vi "Controller Process.vi"(8 "error in (no error)":errorcluster, 11 "View Model":T1) -> (0 "error out":errorcluster)   [LabVIEW 2017]
doc: "The SW component that allows the user to interact with the controls and provides appropriate feedback."
uses:
  Model/Controls/View Model.ctl
  Model/Controls/Shared Model.ctl
  Error Handler/Controls/Error Model.ctl
  Error Handler/Controls/Error Message.ctl
  Error Handler/Controls/Error Type.ctl
  Configuration/Controls/Config Model.ctl
  Configuration/Controls/Config DB Message.ctl
  Configuration/Controls/Config DB Command.ctl
  Configuration/Controls/Config DB Overhead.ctl
  Configuration/Controls/Config DB Record.ctl
  Controls/Controller Model.ctl
  Views/Vehicle Position Simulation View/Controls/Vehicle - Position.ctl
  Controls/Controller Overhead.ctl
  Controls/Controller Wash Step.ctl
  Controls/Controller State.ctl
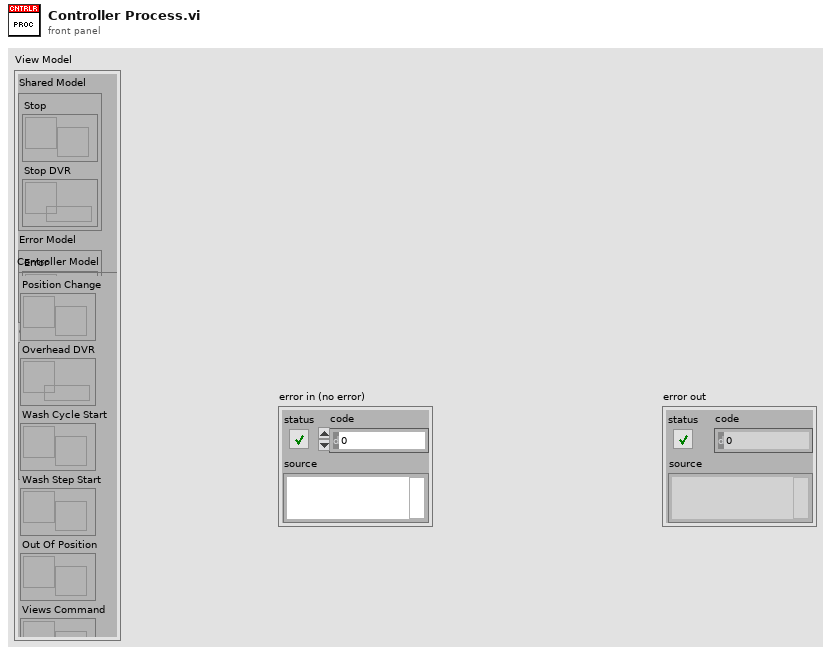
[diagram p1: front panel]
types:
  T1 = typedef "View Model.ctl" = cluster{"Shared Model":T2, "Error Model":T3, "Config Model":T4, "Controller Model":T5}
  T2 = typedef "Shared Model.ctl" = cluster{"Stop":refnum<user-event>, "Stop DVR":refnum<data-value>}
  T3 = typedef "Error Model.ctl" = cluster{"Error":refnum<user-event>}
  T4 = typedef "Config Model.ctl" = cluster{"Config":refnum<user-event>, "Config DVR":refnum<data-value>}
  T5 = typedef "Controller Model.ctl" = cluster{"Position Change":refnum<user-event>, "Overhead DVR":refnum<data-value>, "Wash Cycle Start":refnum<user-event>, "Wash Step Start":refnum<user-event>, "Out Of Position":refnum<user-event>, "Views Command":refnum<user-event>}
  T6 = typedef "Controller State.ctl" = enum16{"Initial", "Wait for Start", "Wash Cycle Start", "Wash Cycle Complete", "Wash Step Start", "Wash Step Execute", "Wash Step Complete", "Wait for Vehicle Position", "Wash Exit", "Wash Abort/Terminate"}
  T7 = typedef "Error Type.ctl" = enum16{"Minor Error", "Wash Cycle Error", "System Error", "Unknown"}
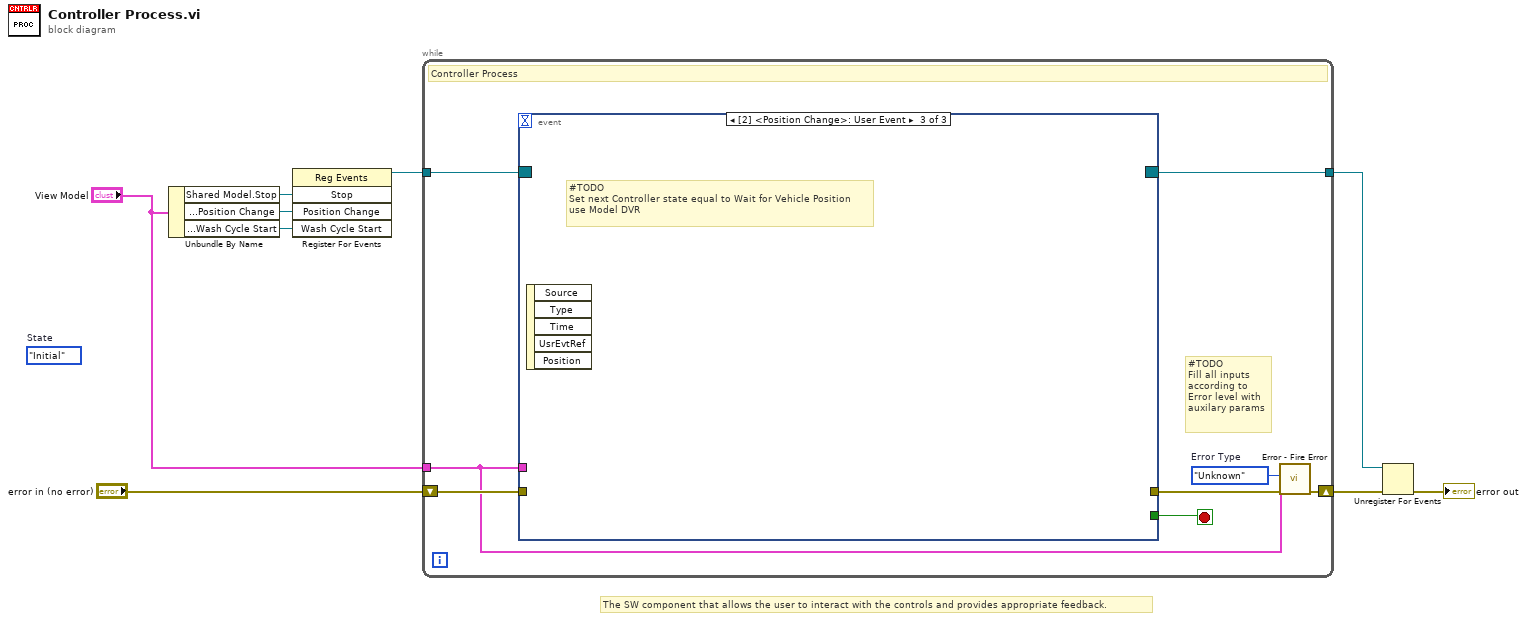
[diagram p0: block diagram]
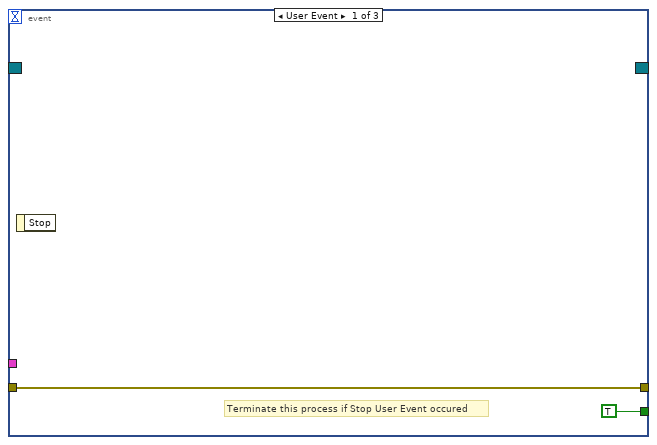
[diagram p2: hidden frame]
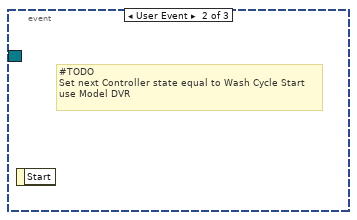
[diagram p3: hidden frame]
diagram:
  (unwired) Controller_State."Initial"  # State
  # "The SW component that allows the user to interact with the controls and provides appropriate feedback."
  n1 = Unbundle By Name("View Model") -> ("Shared Model.Stop"=w9:refnum<user-event>, "Controller Model.Position Change"=w2:refnum<user-event>, "Controller Model.Wash Cycle Start"=w1:refnum<user-event>)
  n2 = register-events(w9, w2, w1) -> (reference out=w8:refnum<event-registration>)  [unwired: 2 in, 1 out]
  n3 = while {
    tunnel: w8 -> [w17]
    shift-right: [w12] -> w6
    shift-left: "error in (no error)" -> [w16]
    tunnel: [w15] -> w4
    tunnel: "View Model" -> [w10]
    stop <- w14 stop-if-true
    w11 = Error_Type."Unknown"  # Error Type
    # "#TODO\nFill all inputs\naccording to \nError level with\nauxilary params"
    # "Controller Process"
    n4 = event shown="[2] <Position Change>: User Event" {
      selector: w17 -> [_ _ _]
      dyn-events: [_ _ _] -> w15
      timeout: _ -> [_ _ _]
      tunnel: w16 -> [w19 _ _]
      tunnel: [w19 _ _] -> w13
      tunnel: w10 -> [_ _ _]
      tunnel: [TRUE _ _] -> w14
      event User Event {
        # "Terminate this process if Stop User Event occured"
        n5 = event-data() -> ()  [unwired: 1 in, 1 out]
      }
      event User Event {
        # "#TODO\nSet next Controller state equal to Wash Cycle Start\nuse Model DVR"
        n6 = event-data() -> ()  [unwired: 1 in, 1 out]
      }
      event User Event {
        # "#TODO\nSet next Controller state equal to Wait for Vehicle Position\nuse Model DVR"
        n7 = event-data() -> ()  [unwired: 1 in, 5 out]
      }
    }
    n8 = call "Error - Fire Error.vi"("error in (no error)"=w13, "Error Type"=w11, "View Model"=w10) -> ("error out"=w12:errorcluster)  [unwired: 7 in, 1 out]
  }
  n9 = Unregister For Events(event registration refnum=w4, error in=w6) -> (error out=→"error out":errorcluster)
